vi "LoadHighscores.vi"(8 "error in (no error)":errorcluster, 11 "Highscore in":refnum<class "Highscore.lvclass">) -> (0 "error out":errorcluster, 3 "Highscore out":refnum<class "Highscore.lvclass">)   [LabVIEW 2019, in "RT_Game.lvlib" / "Highscore.lvclass"]
uses:
  Highscore.lvclass
  HighscoreEntry.ctl
  Highscore.lvclass/Highscore.ctl
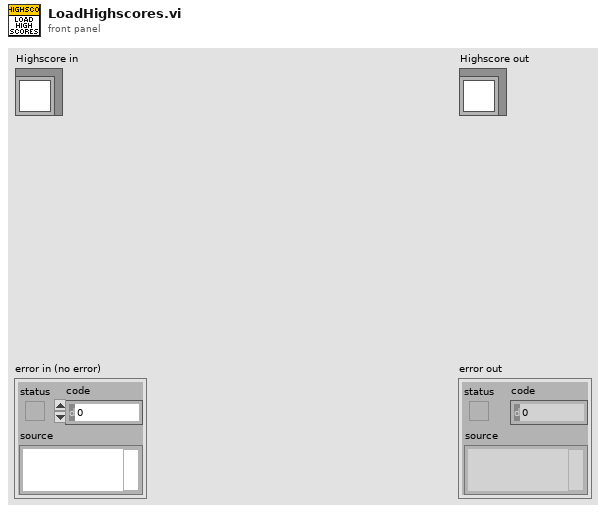
[diagram p1: front panel]
types:
  T1 = typedef "RT_Game.lvlib/Highscore.lvclass/HighscoreEntry.ctl" = cluster{"Name":string, "Score":dbl}
  T2 = enum16{"open", "replace", "create", "open or create", "replace or create", "replace or create with confirmation"}
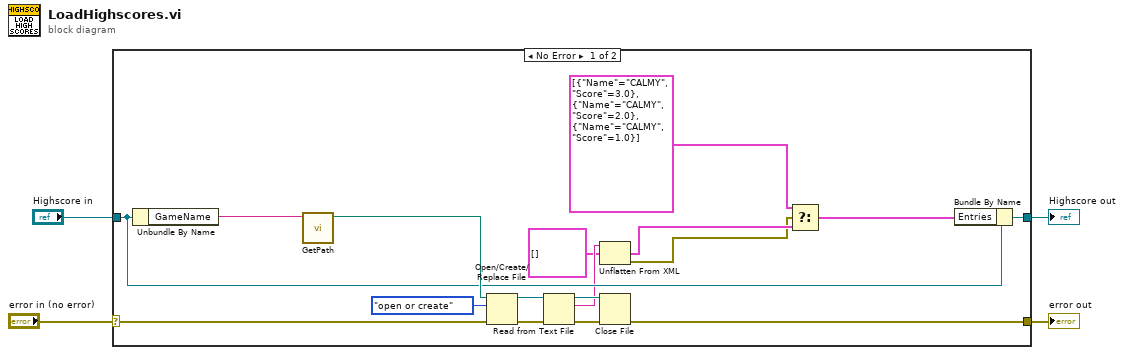
[diagram p0: block diagram]
diagram:
  n1 = case shown="No Error" "error in (no error)" {
    selector: "error in (no error)" -> [w21 w23]
    tunnel: [w13 w23] -> w3
    tunnel: [w9 w22] -> w1
    tunnel: "Highscore in" -> [w18 w22]
    frame No Error {
      n2 = Unbundle By Name(w18) -> ("GameName"=w17:string)
      n3 = call "GetPath.vi"("GameName"=w17) -> ("appended path"=w19:path)  [unwired: 10 in]
      n4 = Open/Create/Replace File(file path (use dialog)=w19, error in=w21, operation (0:open)=T2."open or create") -> (refnum out=w14:refnum<file>, error out=w20:errorcluster)  [unwired: 3 in, 1 out]
      n5 = Read from Text File(file (use dialog)=w14, error in=w20) -> (refnum out=w12:refnum<file>, text=w11:string, error out=w15:errorcluster)  [unwired: 2 in, 1 out]
      n6 = Unflatten From XML(xml string=w11, type=T1[] [] ("Entries")) -> (value=w7:T1[], error out=w5:errorcluster)  [unwired: 1 in]
      n7 = Close File(refnum=w12, error in=w15) -> (error out=w13:errorcluster)  [unwired: 1 out]
      n8 = Select(t=T1[] [{"Name"="CALMY", "Score"=3.0}, {"Name"="CALMY", "Score"=2.0}, {"Name"="CALMY", "Score"=1.0}], s=w5, f=w7) -> (s? t:f=w8:T1[])
      n9 = Bundle By Name(cluster=w18, "Entries"=w8) -> (w9:refnum<class "Highscore.lvclass">)
    }
    frame Error {
    }
  }
  "error out" <- w3
  "Highscore out" <- w1
